vi "DeleteChannels.vi"(8 "error in (no error)":errorcluster, 11 "Item Ref out":T1=18446744073709551615 format="%.0x") -> (0 "error out":errorcluster, 3 "Parent Ref out":T1 format="%.0x")   [LabVIEW 2017]
uses:
  <vilib>/NI Veristand/Custom Device API/Custom Device Item Ref.ctl
  Global_VS_ref.vi
  <vilib>/NI Veristand/Custom Device API/Custom Device API.lvlib
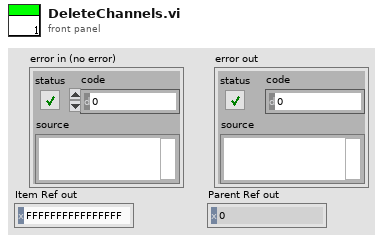
[diagram p1: front panel]
types:
  T1 = typedef "Custom Device API.lvlib/Custom Device Item Ref.ctl" = u64
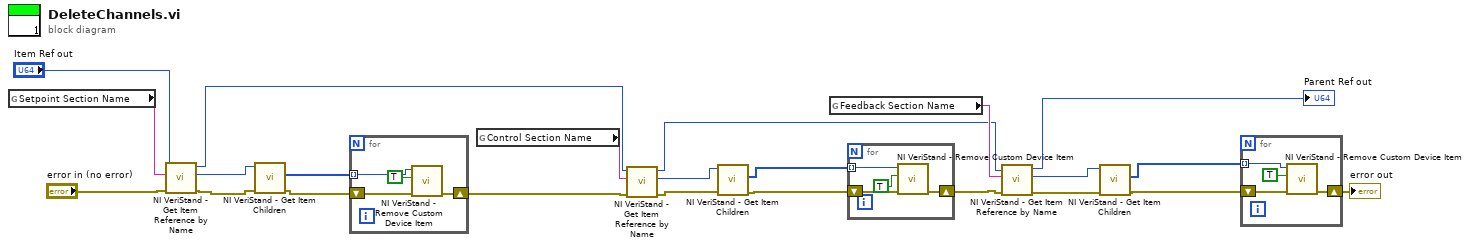
[diagram p0: block diagram]
diagram:
  n1 = global read "Global_VS_ref.vi" "Setpoint Section Name"() -> (w22:string)
  n2 = call <vilib>:"NI VeriStand - Get Item Reference by Name.vi"("error in (no error)"="error in (no error)", "Item Name"=w22, "Parent Ref in"="Item Ref out") -> ("error out"=w10:errorcluster, "Item Ref"=w12:T1, "Parent Ref out"=w17:T1)  [unwired: 5 in, 1 out]
  n3 = call <vilib>:"NI VeriStand - Get Item Children.vi"("error in (no error)"=w10, "Item Ref in"=w12) -> ("error out"=w9:errorcluster, "Child Refs"=w11:T1[])  [unwired: 6 in, 2 out]
  n4 = for {
    tunnel: w11 -> [w24] mode=indexing
    shift-right: [w25] -> w16
    shift-left: w9 -> [w26]
    n5 = call <vilib>:"NI VeriStand - Remove Custom Device Item.vi"("error in (no error)"=w26, "Force Delete (F)"=TRUE, "Item Ref in"=w24) -> ("error out"=w25:errorcluster)  [unwired: 7 in, 1 out]
  }
  n6 = global read "Global_VS_ref.vi" "Control Section Name"() -> (w21:string)
  n7 = call <vilib>:"NI VeriStand - Get Item Reference by Name.vi"("error in (no error)"=w16, "Item Name"=w21, "Parent Ref in"=w17) -> ("error out"=w7:errorcluster, "Item Ref"=w8:T1, "Parent Ref out"=w14:T1)  [unwired: 5 in, 1 out]
  n8 = call <vilib>:"NI VeriStand - Get Item Children.vi"("error in (no error)"=w7, "Item Ref in"=w8) -> ("error out"=w6:errorcluster, "Child Refs"=w5:T1[])  [unwired: 6 in, 2 out]
  n9 = global read "Global_VS_ref.vi" "Feedback Section Name"() -> (w20:string)
  n10 = for {
    shift-right: [w30] -> w15
    shift-left: w6 -> [w29]
    tunnel: w5 -> [w28] mode=indexing
    n11 = call <vilib>:"NI VeriStand - Remove Custom Device Item.vi"("error in (no error)"=w29, "Force Delete (F)"=TRUE, "Item Ref in"=w28) -> ("error out"=w30:errorcluster)  [unwired: 7 in, 1 out]
  }
  n12 = call <vilib>:"NI VeriStand - Get Item Reference by Name.vi"("error in (no error)"=w15, "Item Name"=w20, "Parent Ref in"=w14) -> ("error out"=w3:errorcluster, "Item Ref"=w4:T1, "Parent Ref out"=→"Parent Ref out":T1)  [unwired: 5 in, 1 out]
  n13 = call <vilib>:"NI VeriStand - Get Item Children.vi"("error in (no error)"=w3, "Item Ref in"=w4) -> ("error out"=w2:errorcluster, "Child Refs"=w1:T1[])  [unwired: 6 in, 2 out]
  n14 = for {
    shift-right: [w35] -> w23
    shift-left: w2 -> [w33]
    tunnel: w1 -> [w32] mode=indexing
    n15 = call <vilib>:"NI VeriStand - Remove Custom Device Item.vi"("error in (no error)"=w33, "Force Delete (F)"=TRUE, "Item Ref in"=w32) -> ("error out"=w35:errorcluster)  [unwired: 7 in, 1 out]
  }
  "error out" <- w23
